vi "Pre-Build Action.vi"(6 "Top Level/Always Included VIs":path[](array[path]), 7 "Main Destination Path":path, 9 "Target Name":string, 10 "Build Specification Name":string, 11 "Project Path":path) -> (0 "error out":errorcluster)   [LabVIEW 2021]
panel:
  out "UID":i32
  out "Class Name":string
  out "error out 2":errorcluster
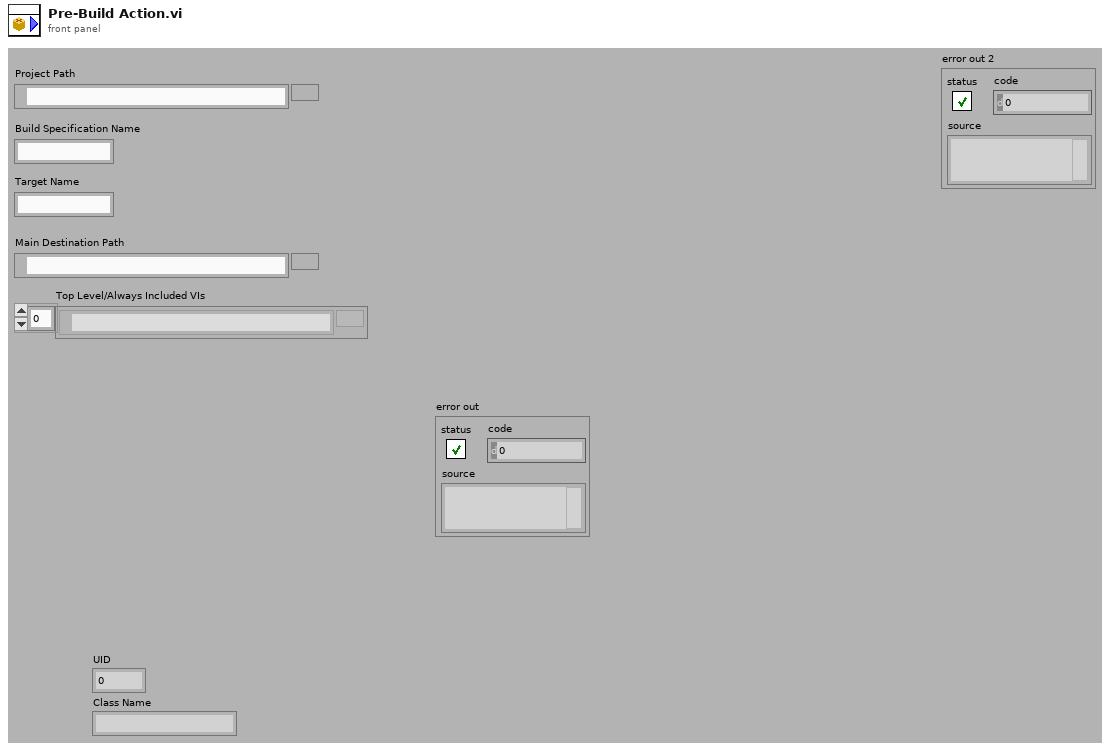
[diagram p1: front panel]
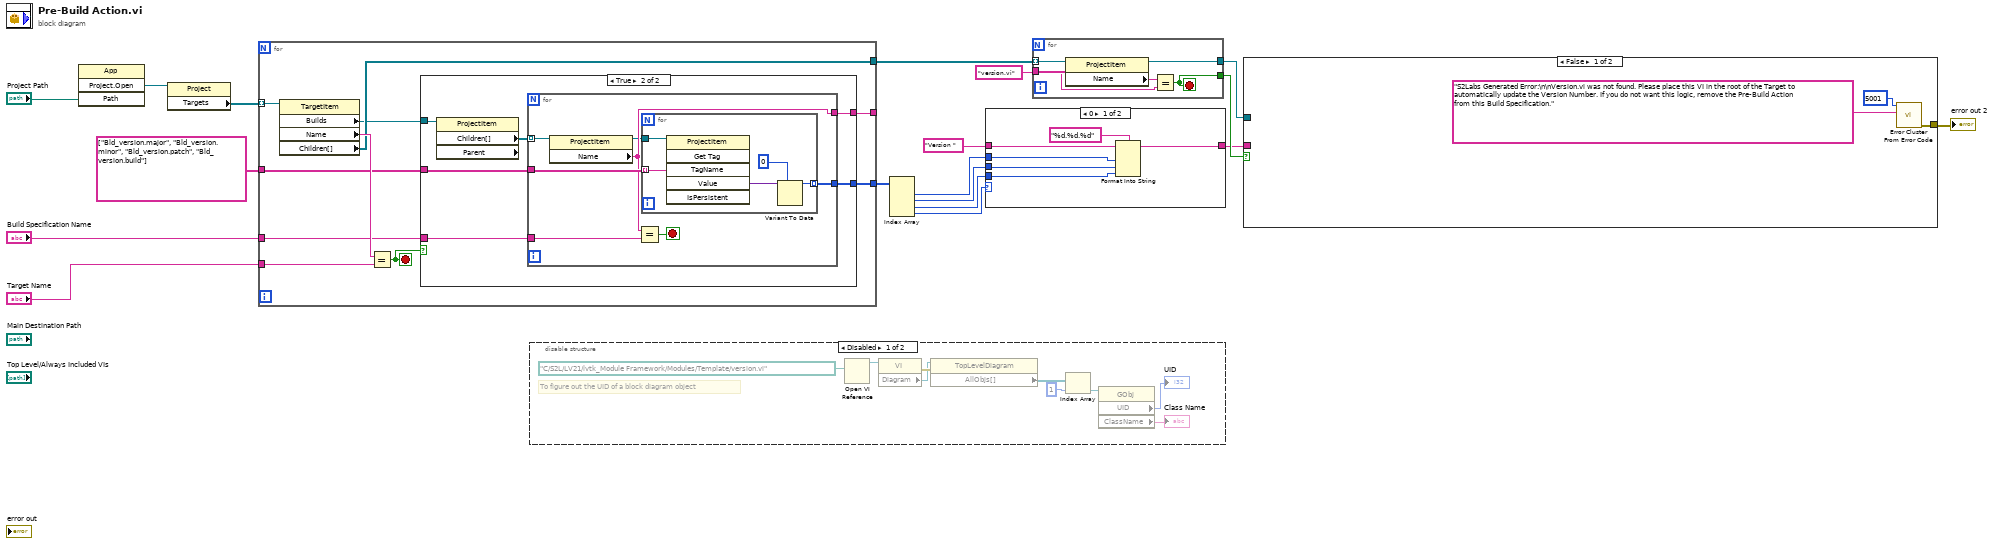
[diagram p0: block diagram]
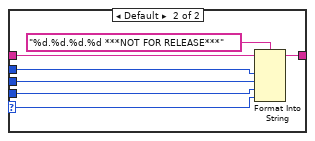
[diagram p3: hidden frame]
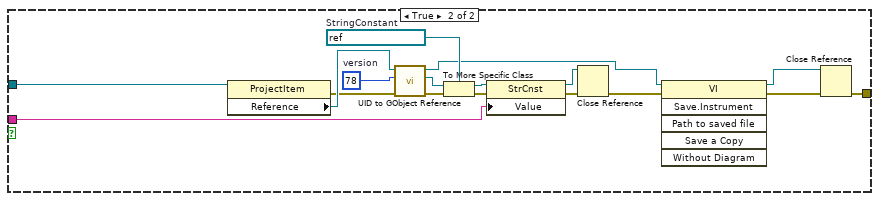
[diagram p5: hidden frame]
diagram:
  n1 = invoke class="App" method="Project.Open"("Path"="Project Path") -> ("Project:Open"=w15:refnum<vi>)  [unwired: 3 in, 3 out]
  n2 = property class="Project"(reference=w15) -> ("Targets"=w14:refnum<vi>[])  [unwired: 1 in, 2 out]
  n3 = for {
    tunnel: w14 -> [w28] mode=indexing
    tunnel: "Target Name" -> [w26]
    tunnel: "Build Specification Name" -> [w25]
    tunnel: string[] ["Bld_version.major", "Bld_version.minor", "Bld_version.patch", "Bld_version.build"] -> [w24]
    tunnel: [w23] -> w12
    tunnel: [w21] -> _
    tunnel: [w20] -> w17
    stop <- w22 stop-if-true
    n4 = property class="TargetItem"(reference=w28) -> ("Builds"=w19:refnum<vi>, "Name"=w27:string, "Children[]"=w20:refnum<vi>[])  [unwired: 1 in, 2 out]
    n5 = Equal?(x=w27, y=w26) -> (x = y?=w22:bool)
    n6 = case shown="True" w22 {
      tunnel: w19 -> [_ w34]
      tunnel: w25 -> [_ w32]
      tunnel: w24 -> [_ w31]
      tunnel: [_ w30] -> w23
      tunnel: [_ w29] -> w21
      frame False {
      }
      frame True {
        n7 = property class="ProjectItem" props=["Children[]", "Parent"](reference=w34) -> ("Children[]"=w33:refnum<vi>[])  [unwired: 1 in, 3 out]
        n8 = for {
          tunnel: w33 -> [w41] mode=indexing
          tunnel: w32 -> [w40]
          tunnel: w31 -> [w38]
          tunnel: [w37] -> w30
          tunnel: [w36] -> w29
          stop <- w39 stop-if-true
          n9 = property class="ProjectItem"(reference=w41) -> (reference out=w35:refnum<vi>, "Name"=w36:string)  [unwired: 1 in, 1 out]
          n10 = Equal?(x=w36, y=w40) -> (x = y?=w39:bool)
          n11 = for {
            tunnel: w35 -> [w46]
            tunnel: w38 -> [w45] mode=indexing
            tunnel: [w42] -> w37 mode=indexing
            n12 = invoke class="ProjectItem" method="Get Tag"(reference=w46, "TagName"=w45) -> ("Value"=w44:variant)  [unwired: 4 in, 5 out]
            n13 = Variant To Data(type=0, Variant=w44) -> (data=w42:i32)  [unwired: 1 in, 1 out]
          }
        }
      }
    }
  }
  n14 = disable-structure shown="Disabled" {
    frame Disabled {
      # "To figure out the UID of a block diagram object"
      n15 = Open VI Reference(vi path=path "C:/S2L/LV21/lvtk_Module Framework/Modules/Template/version.vi") -> (vi reference=w52:refnum<vi>)  [unwired: 5 in, 1 out]
      n16 = property class="VI"(reference=w52) -> (error out=w54:errorcluster, "Diagram"=w53:refnum<vi>)  [unwired: 1 in, 1 out]
      n17 = property class="TopLevelDiagram"(reference=w53, error in=w54) -> ("AllObjs[]"=w51:refnum<vi>[])  [unwired: 2 out]
      n18 = Index Array(array=w51, index=1) -> (element=w49:refnum<vi>)
      n19 = property class="GObj"(reference=w49) -> ("UID"=→"UID":i32, "ClassName"=→"Class Name":string)  [unwired: 1 in, 2 out]
    }
    frame Enabled {
    }
  }
  n20 = Index Array(array=w12) -> (element #1=w11:i32, element #2=w10:i32, element #3=w9:i32, element #4=w7:i32)  [unwired: 4 in]
  n21 = case shown="0" w7 {
    selector: w7 -> [_ w64]
    tunnel: w11 -> [w60 w67]
    tunnel: w10 -> [w59 w66]
    tunnel: w9 -> [w58 w65]
    tunnel: [w57 w63] -> w5
    tunnel: "Version " -> [w56 w62]
    frame 0 {
      n22 = Format Into String(format string="%d.%d.%d", initial string=w56, w60, w59, w58) -> (resulting string=w57:string)  [unwired: 1 in, 1 out]
    }
    frame Default {
      n23 = Format Into String(format string="%d.%d.%d.%d ***NOT FOR RELEASE***", initial string=w62, w67, w66, w65, w64) -> (resulting string=w63:string)  [unwired: 1 in, 1 out]
    }
  }
  n24 = for {
    tunnel: w17 -> [w73] mode=indexing
    tunnel: "version.vi" -> [w72]
    tunnel: [w70] -> w16
    tunnel: [w69] -> w8
    stop <- w69 stop-if-true
    n25 = property class="ProjectItem"(reference=w73) -> (reference out=w70:refnum<vi>, "Name"=w71:string)  [unwired: 1 in, 1 out]
    n26 = Equal?(x=w71, y=w72) -> (x = y?=w69:bool)
  }
  n27 = case shown="False" w8 {
    tunnel: w5 -> [_ w93]
    tunnel: w16 -> [_ w92]
    tunnel: [w74 w77] -> w6
    frame False {
      n28 = call <vilib>:"Error Cluster From Error Code.vi"("error message (\"\")"="S2Labs Generated Error:\n\nVersion.vi was not found. Please place this VI in the root of the Target to automatically update the Version Number. If you do not want this logic, remove the Pre-Build Action from this Build Specification." ("message"), "error code (0)"=5001) -> ("error out"=w74:errorcluster)  [unwired: 7 in]
    }
    frame True {
      w85 = 78  # version
      w84 = refnum<vi> refnum  # StringConstant
      n29 = property class="ProjectItem"(reference=w92) -> (error out=w82:errorcluster, "Reference"=w83:refnum<vi>)  [unwired: 1 in, 1 out]
      n30 = call <vilib>:"UID to GObject Reference.vi"("error in (no error)"=w82, "UID"=w85, "Owning VI"=w83) -> ("error out"=w91:errorcluster, "GObject"=w86:refnum<vi>, "dup Owning VI"=w80:refnum<vi>)  [unwired: 6 in]
      n31 = To More Specific Class(target class=w84, reference=w86, error in=w91) -> (specific class reference=w87:refnum<vi>, error out=w90:errorcluster)
      n32 = property class="StrCnst"(reference=w87, error in=w90, "Value"=w93) -> (reference out=w89:refnum<vi>, error out=w88:errorcluster)
      n33 = Close Reference(reference=w89, error in (no error)=w88) -> (error out=w81:errorcluster)
      n34 = invoke class="VI" method="Save.Instrument"(reference=w80, error in=w81) -> (reference out=w79:refnum<vi>, error out=w78:errorcluster)  [unwired: 4 in, 4 out]
      n35 = Close Reference(reference=w79, error in (no error)=w78) -> (error out=w77:errorcluster)
    }
  }
  "error out 2" <- w6
